vi "fgt detect.vi"(8 "error in (no error)":errorcluster) -> (0 "error out":errorcluster, 2 "type out":T1[](array[typedef]), 3 "SN out":u16[](array[numeric]))   [LabVIEW 2020, in "fgt_SDK.lvlib"]
doc: "Detects all connected Fluigent instrument(s), return their serial number and type"
uses:
  fgt_SDK.lvlib
  TypeDefs/fgt_INSTRUMENT_TYPE.ctl
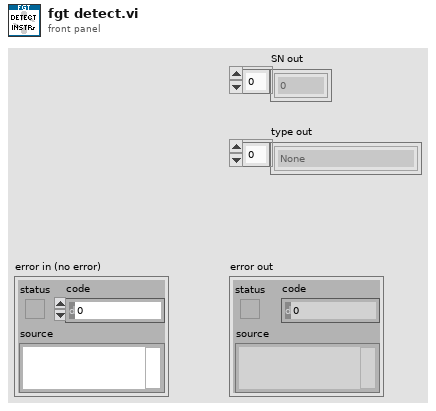
[diagram p1: front panel]
types:
  T1 = typedef "fgt_SDK.lvlib/fgt_INSTRUMENT_TYPE.ctl" = enum32{"None", "MFCS", "MFCS_EZ", "FRP", "LineUP", "IPS"}
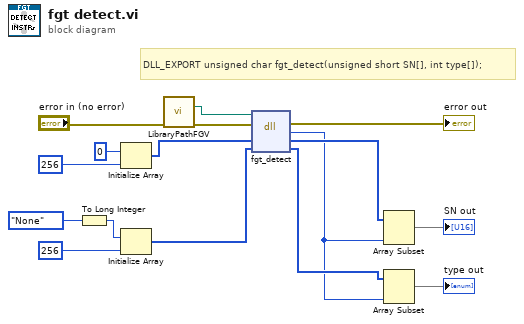
[diagram p0: block diagram]
diagram:
  # "DLL_EXPORT unsigned char fgt_detect(unsigned short SN[], int type[]);"
  n1 = To Long Integer(number=fgt_INSTRUMENT_TYPE."None" ("fgt_INSTRUMENT_TYPE")) -> (32bit integer=w5:i32)
  n2 = Initialize Array(u16 0 ("element"), 256 ("dimension size")) -> (w8:u16[])
  n3 = Initialize Array(w5, 256 ("dimension size")) -> (w7:i32[])
  n4 = call "LibraryPathFGV.vi"("error in (no error)"="error in (no error)") -> ("Path Out"=w3:path, "error out"=w2:errorcluster)  [unwired: 13 in]
  n5 = dll-call lib="C:/Workspace/fgt-SDK/LabVIEW/dlls/fgt_SDK_*.*" fn="fgt_detect"(path in=w3, error in=w2, "SN"=w8, "type"=w7) -> (error out=→"error out":errorcluster, "return type"=w4:u8, "SN"=w15:u16[], "type"=w13:i32[])  [unwired: 1 in, 1 out]
  n6 = Array Subset(array=w15, length=w4) -> (→"SN out":u16[])  [unwired: 1 in]
  n7 = Array Subset(array=w13, length=w4) -> (→"type out":i32[])  [unwired: 1 in]
